vi "decode btr.vi"(10 "clock frequency (8 MHz)":u8=8, 11 "btr":u16 format="%04x") -> (1 "sample point [%]":dbl, 2 "triple sampling":bool, 3 "bitrate parameters":T1, 4 "btr1":u8 format="%02x", 5 "duration of single time quantum [s]":dbl format="%#_6p", 6 "btr0":u8 format="%02x", 7 "num of time quanta per bit":u16)   [LabVIEW 2024, in "atsj peakcan basic.lvlib"]
doc: "Converts a <b>btr</b> (Bus Timing Register) value into the corresponding <b>bitrate parameters</b>.\n\nCopyright (c) 2025 ATSJ (www.atsj.eu)"
uses:
  atsj peakcan basic.lvlib
  bitrate parameters.ctl
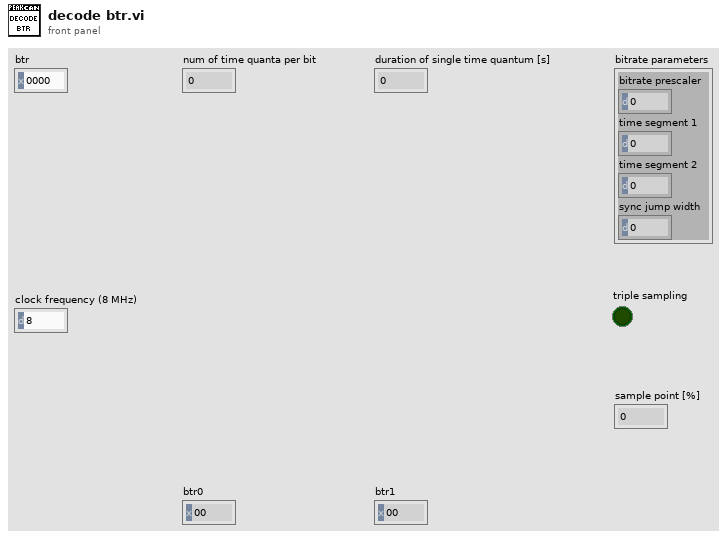
[diagram p1: front panel]
types:
  T1 = typedef "atsj peakcan basic.lvlib/bitrate parameters.ctl" = cluster{"bitrate prescaler":u16, "time segment 1":u16, "time segment 2":u16, "sync jump width":u16}
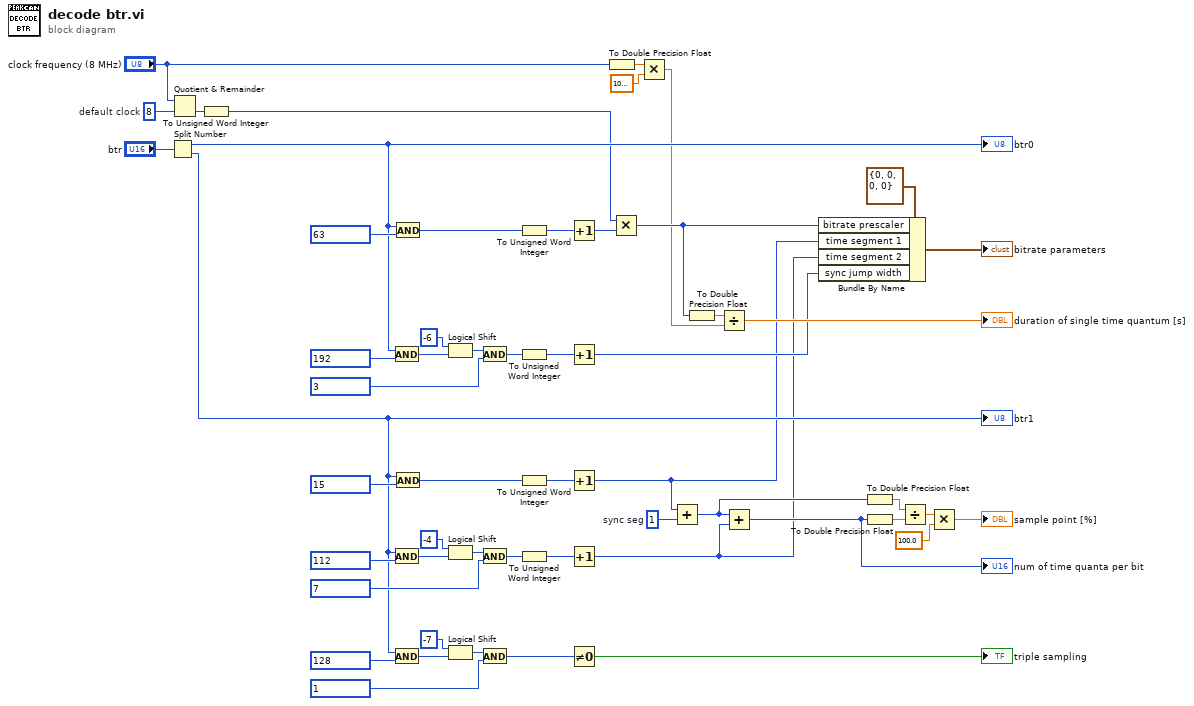
[diagram p0: block diagram]
diagram:
  w20 = u16 1  # sync seg
  w29 = u8 8  # default clock
  n1 = Split Number(x="btr") -> (hi(x)=w49:u8, lo(x)=w30:u8)
  "btr0" <- w49
  "btr1" <- w30
  n2 = Quotient & Remainder(x="clock frequency (8 MHz)", y=w29) -> (floor(x/y)=w28:u8)  [unwired: 1 out]
  n3 = To Unsigned Word Integer(number=w28) -> (unsigned 16bit integer=w1:u16)
  n4 = And(x=w49, y=u8 192) -> (x .and. y?=w45:u8)
  n5 = And(x=w30, y=u8 112) -> (x .and. y?=w42:u8)
  n6 = And(x=w30, y=u8 128) -> (x .and. y?=w31:u8)
  n7 = And(x=w49, y=u8 63) -> (x .and. y?=w52:u8)
  n8 = And(x=w30, y=u8 15) -> (x .and. y?=w37:u8)
  n9 = Logical Shift(y=i16 -6, x=w45) -> (x << y=w47:u8)
  n10 = Logical Shift(y=i16 -4, x=w42) -> (x << y=w40:u8)
  n11 = Logical Shift(y=i16 -7, x=w31) -> (x << y=w33:u8)
  n12 = And(x=w47, y=u8 3) -> (x .and. y?=w44:u8)
  n13 = And(x=w40, y=u8 7) -> (x .and. y?=w43:u8)
  n14 = And(x=w33, y=u8 1) -> (x .and. y?=w27:u8)
  n15 = To Unsigned Word Integer(number=w52) -> (unsigned 16bit integer=w10:u16)
  n16 = To Unsigned Word Integer(number=w44) -> (unsigned 16bit integer=w9:u16)
  n17 = To Unsigned Word Integer(number=w37) -> (unsigned 16bit integer=w8:u16)
  n18 = To Unsigned Word Integer(number=w43) -> (unsigned 16bit integer=w7:u16)
  n19 = Increment(x=w10) -> (x+1=w51:u16)
  n20 = Increment(x=w9) -> (x+1=w11:u16)
  n21 = Increment(x=w8) -> (x+1=w6:u16)
  n22 = Increment(x=w7) -> (x+1=w2:u16)
  n23 = Not Equal To 0?(x=w27) -> (x != 0?=→"triple sampling":bool)
  n24 = To Double Precision Float(number="clock frequency (8 MHz)") -> (double precision float=w24:dbl)
  n25 = Multiply(x=w1, y=w51) -> (x*y=w13:u16)
  n26 = Multiply(x=w24, y=1000000.0) -> (x*y=w12:dbl)
  n27 = Add(x=w6, y=w20) -> (x+y=w3:u16)
  n28 = To Double Precision Float(number=w13) -> (double precision float=w22:dbl)
  n29 = Divide(x=w22, y=w12) -> (x/y=→"duration of single time quantum [s]":dbl)
  n30 = Add(x=w3, y=w2) -> (x+y=w19:u16)
  "num of time quanta per bit" <- w19
  n31 = Bundle By Name(cluster=T1 {"bitrate prescaler"=0, "time segment 1"=0, "time segment 2"=0, "sync jump width"=0}, "bitrate prescaler"=w13, "time segment 1"=w6, "time segment 2"=w2, "sync jump width"=w11) -> (→"bitrate parameters":T1)
  n32 = To Double Precision Float(number=w3) -> (double precision float=w17:dbl)
  n33 = To Double Precision Float(number=w19) -> (double precision float=w18:dbl)
  n34 = Divide(x=w17, y=w18) -> (x/y=w4:dbl)
  n35 = Multiply(x=w4, y=100.0) -> (x*y=→"sample point [%]":dbl)
